vi "detector_set_integration_time_seconds.vi"(8 "error in (no error)":errorcluster, 10 "integration time (seconds)":dbl, 11 "tt20 in":refnum<class "tt20.lvclass">) -> (0 "error out":errorcluster, 3 "tt20 out":refnum<class "tt20.lvclass">)   [LabVIEW 2015, in "tt20.lvclass"]
uses:
  tt20.lvclass
  tt20.lvclass/tt20.ctl
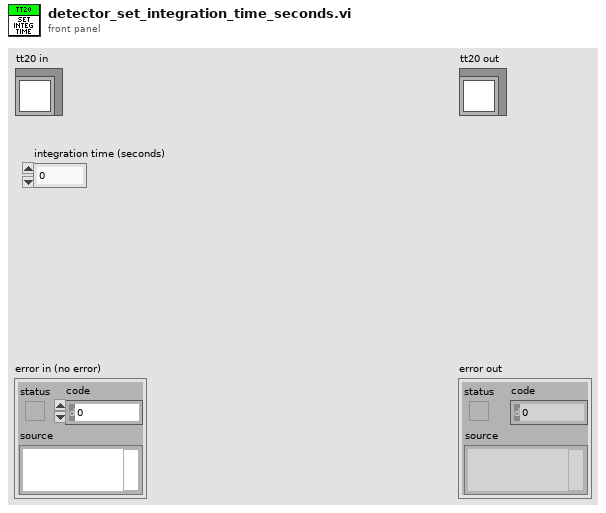
[diagram p1: front panel]
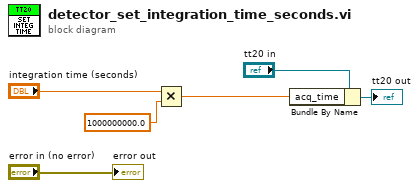
[diagram p0: block diagram]
diagram:
  n1 = Multiply(x="integration time (seconds)", y=1000000000.0) -> (x*y=w3:dbl)
  n2 = Bundle By Name(cluster="tt20 in", "acq_time"=w3) -> (→"tt20 out":refnum<class "tt20.lvclass">)
  "error out" <- "error in (no error)"
